vi "ConfigureCounters.vi"(8 "error in (no error)":errorcluster, 11 "IntanElectrophysiology in":refnum<class "IntanElectrophysiology.lvclass">) -> (0 "error out":errorcluster, 3 "IntanElectrophysiology out":refnum<class "IntanElectrophysiology.lvclass">)   [LabVIEW 2014, in "IntanElectrophysiology.lvclass"]
uses:
  IntanElectrophysiology.lvclass
  IntanElectrophysiology.lvclass/IntanElectrophysiology.ctl
panel:
  in  "Intan Clock to Single Pulse":tag="/Dev1/PFI15"
  in  "Periodic AI Trigger":tag="/Dev1/PFI8"
  in  "Divide by N Counter":tag="Dev1/ctr7"
  in  "Single Pulse Duration":dbl=1e-05 format="%.6f"
  in  "AI Start Trigger":tag="/Dev1/PFI12"
  in  "Single Pulse Counter":tag="Dev1/ctr6"
  in  "Divide By N":dbl=300000.0 format="%.6f"
  in  "Intan Clock to Divide by N":tag="/Dev1/PFI11"
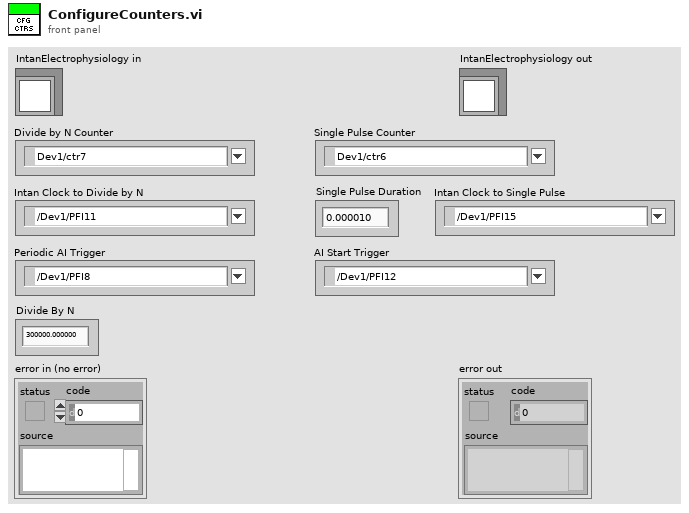
[diagram p1: front panel]
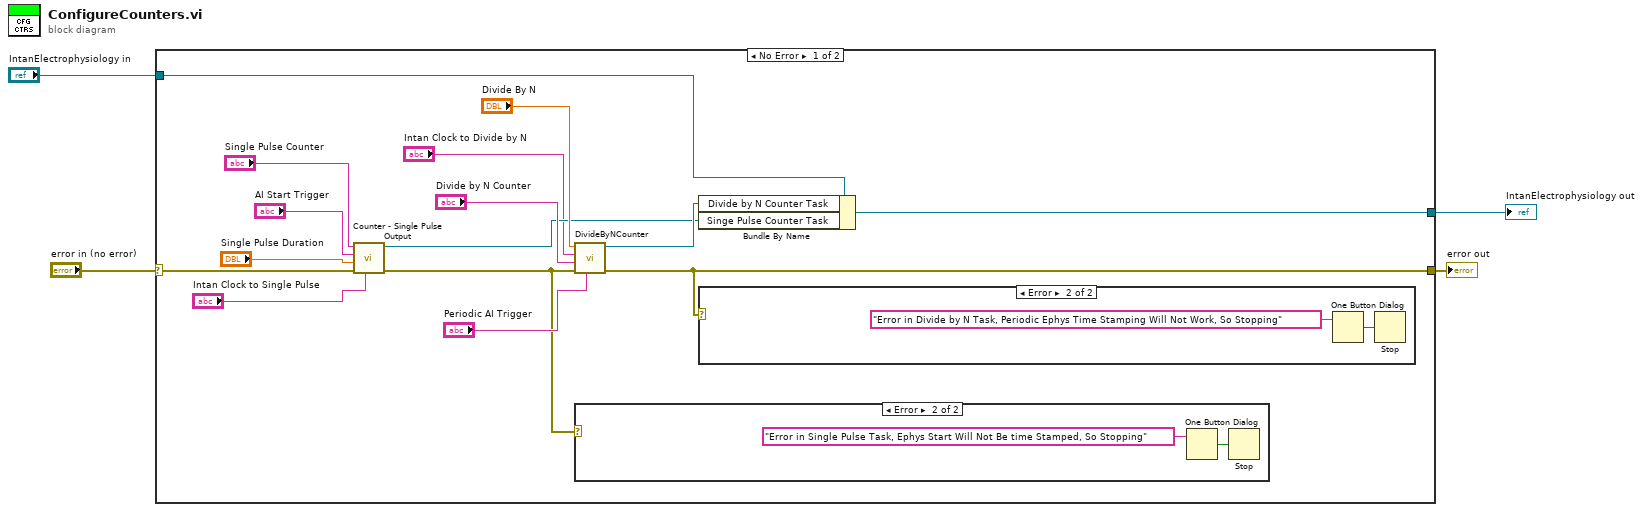
[diagram p0: block diagram]
diagram:
  n1 = case shown="No Error" "error in (no error)" {
    selector: "error in (no error)" -> [w15 w25]
    tunnel: [w11 w25] -> w3
    tunnel: [w7 w24] -> w1
    tunnel: "IntanElectrophysiology in" -> [w10 w24]
    frame No Error {
      n2 = call "Counter - Single Pulse Output.vi"("Digital Trigger Source"="Intan Clock to Single Pulse", "error in"=w15, "Pulse Duration"="Single Pulse Duration", "Output Terminal"="AI Start Trigger", "Counter"="Single Pulse Counter") -> ("error out"=w12:errorcluster, "task out"=w8:refnum<k21>)  [unwired: 5 in]
      n3 = call "DivideByNCounter.vi"("Output Terminal"="Periodic AI Trigger", "error in"=w12, "Counter"="Divide by N Counter", "Input Terminal"="Intan Clock to Divide by N", "Divide By N"="Divide By N") -> ("error out"=w11:errorcluster, "task out"=w9:refnum<k21>)  [unwired: 5 in]
      n4 = case shown="Error" w12 {
        frame No Error {
        }
        frame Error {
          n5 = One Button Dialog(message="Error in Single Pulse Task, Ephys Start Will Not Be time Stamped, So Stopping") -> (true=w22:bool)  [unwired: 1 in]
          n6 = Stop(stop? (T)=w22) -> ()
        }
      }
      n7 = Bundle By Name(cluster=w10, "Divide by N Counter Task"=w9, "Singe Pulse Counter Task"=w8) -> (w7:refnum<class "IntanElectrophysiology.lvclass">)
      n8 = case shown="Error" w11 {
        frame No Error {
        }
        frame Error {
          n9 = One Button Dialog(message="Error in Divide by N Task, Periodic Ephys Time Stamping Will Not Work, So Stopping") -> (true=w20:bool)  [unwired: 1 in]
          n10 = Stop(stop? (T)=w20) -> ()
        }
      }
    }
    frame Error {
    }
  }
  "error out" <- w3
  "IntanElectrophysiology out" <- w1
